vi "BluePlot Main.vi"(10 "Init options":T6={"UI visible?"=FALSE, "Update rate (ms)"=250, "visible sidebar?"=FALSE, "time to plot (init)"=600.0, "time to plot (max)"=inf, "config file start path"=path ""} {"time to plot (init)" format="%<%H:%M:%S>t"}, 11 "BluePlotHandle":refnum<class "BluePlotHandle.lvclass">) -> ()   [LabVIEW 2021, in "BluePlot.lvlib"]
uses:
  BluePlot.lvlib
  TypeDefs/Plot top row.ctl
  Classes/BluePlotHandle/BluePlotHandle.lvclass
  Classes/BluePlotHandle/SubVIs/Init Options.ctl
  TypeDefs/plot load data V2.ctl
  TypeDefs/plot properties V2.ctl
  TypeDefs/plot attributes V2.ctl
  TypeDefs/Plot scale axis properties.ctl
  TypeDefs/Plot general properties.ctl
  TypeDefs/plot event struc data.ctl
  TypeDefs/Plot active mode.ctl
  TypeDefs/Plot UI references.ctl
  TypeDefs/plot while loop data.ctl
  Classes/BluePlotHandle/BluePlotHandle.lvclass/BluePlotHandle.ctl
  SubVIs/autocomplete string/autocomplete key focus states.ctl
  TypeDefs/load config mode.ctl
  <vilib>/Utility/miscctls.llb/LVPointTypeDef.ctl
  TypeDefs/plot handle queue data.ctl
  TypeDefs/Plot QSM action.ctl
  <vilib>/Futures/Futures/Promise/Promise.lvclass
  TypeDefs/Save 1PLOT config.ctl
  <userlib>/Blue Origin/BlueSerialization/BlueSerializer/BlueSerializer.lvclass
  <userlib>/Blue Origin/BlueJSONTextSerializer/Classes/BlueJSONTextSerializer/BlueJSONTextSerializer.lvclass
  C:/Program Files/National Instruments/LabVIEW 2021/user.lib/Blue Origin/BlueSerialization/BlueSerializer/BlueSerializer.lvclass
panel:
  in  "Save 1PLOT (spoof)":bool
  in  "Load 1PLOT (spoof)":bool
  in  "Open Settings (spoof)":bool
  in  "clear plot config":bool
  in  "Load Plot config":T1={"plots"=[], "X-axis"={"Name Label.Text"="", "Style"=0, "Tick Colors:Minor Tick Color"=0, "Tick Colors:Tick Color"=0, "Marker Colors:Text Color"=0, "Grid Colors:Major Color"=0, "Grid Colors:Minor Color"=0, "Mapping Mode"=0, "Flipped"=FALSE, "Name Label.Visible"=FALSE, "Name Label.Text Colors:Text Color"=0, "Scale Fit"=0, "Editable"=FALSE, "Range:Maximum"=0.0, "Range:Minimum"=0.0, "Offset and Multiplier:Multiplier"=0.0, "Offset and Multiplier:Offset"=0.0, "Name Label.Font:Size"=0, "Marker.Font:Size"=0, "Uniform Marker Spacing?"=TRUE, "Format String"=""}, "Y-axes"=[], "General"={"Title"="", "Time to Plot"=1800.0, "Title.Visible"=FALSE, "Sidebar.Visible"=FALSE, "Plot Area:Colors:BG Color"=0}} {"General"."Time to Plot" format="%<%M:%S>t"}
  in  "Tab":enum32{"Page 1"}(tab)
  in  "Add row":bool
  in  "Time to Plot":dbl=1800.0 format="%<%H:%M:%S>t"
  in  "Title Visible?":bool
  in  "Splitter locked?":bool
  in  "Erase Plot":bool
  in  "Open Settings":bool
  in  "Save 1PLOT":bool
  in  "Load 1PLOT":bool
  out "Numerics":dbl[](array[numeric])
  in  "Scrollbar":i32(c297)
  in  "spoof1":T7(graph)
  out "dummy":bool
  in  "visible?":bool
  in  "top array":T8[](array[typedef])
  in  "Shutdown":bool
  in  "Title":string="Title"
  in  "visible sidebar?":bool
  out "Plot":cluster{"Timestamps":dbl[], "Data":dbl[]}[](graph)
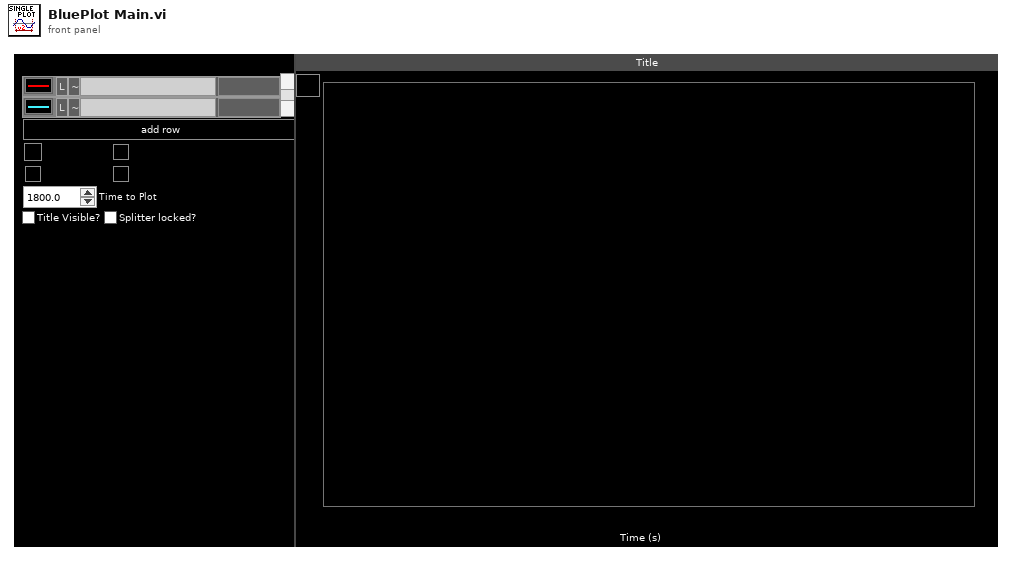
[diagram p1: front panel]
types:
  T1 = typedef "BluePlot.lvlib/plot load data V2.ctl" = cluster{"plots":T2[], "X-axis":T4, "Y-axes":T4[], "General":T5}
  T2 = typedef "BluePlot.lvlib/plot properties V2.ctl" = cluster{"attributes":T3, "Numeric":dbl, "Flatline?":bool}
  T3 = typedef "BluePlot.lvlib/plot attributes V2.ctl" = cluster{"Plot Color":u32, "Point Style":u8, "Line Style":u8, "Plot Interpolation":u8, "Line Width":u8, "Bar Plot Style":u8, "Fill To":i16, "X Scale Index":u32, "Y Scale Index":u32, "Anti-aliased":bool, "Label Format":u8, "Digital Transition Type":u8, "Digital Transition Location":u8, "Digital Line Style":u8, "Fill/Point Color":u32, "Plot Name":string, "Visible":bool}
  T4 = typedef "BluePlot.lvlib/Plot scale axis properties.ctl" = cluster{"Name Label.Text":string, "Style":u8, "Tick Colors:Minor Tick Color":u32, "Tick Colors:Tick Color":u32, "Marker Colors:Text Color":u32, "Grid Colors:Major Color":u32, "Grid Colors:Minor Color":u32, "Mapping Mode":u8, "Flipped":bool, "Name Label.Visible":bool, "Name Label.Text Colors:Text Color":u32, "Scale Fit":u8, "Editable":bool, "Range:Maximum":dbl, "Range:Minimum":dbl, "Offset and Multiplier:Multiplier":dbl, "Offset and Multiplier:Offset":dbl, "Name Label.Font:Size":u32, "Marker.Font:Size":u32, "Uniform Marker Spacing?":bool, "Format String":string}
  T5 = typedef "BluePlot.lvlib/Plot general properties.ctl" = cluster{"Title":string, "Time to Plot":dbl, "Title.Visible":bool, "Sidebar.Visible":bool, "Plot Area:Colors:BG Color":u32}
  T6 = typedef "BluePlot.lvlib/BluePlotHandle.lvclass/Init Options.ctl" = cluster{"UI visible?":bool, "Update rate (ms)":u32, "visible sidebar?":bool, "time to plot (init)":dbl, "time to plot (max)":dbl, "config file start path":path}
  T7 = cluster{cluster{"Time Stamp":dbl, "Data Value":dbl}[]}[]
  T8 = typedef "BluePlot.lvlib/Plot top row.ctl" = cluster{"PID":string, "index":i32, "PID color":u32, "right axis?":bool, "Flatline?":bool, "Numeric color":u32, "Data":string, "Flat":string}
  T9 = typedef "BluePlot.lvlib/plot while loop data.ctl" = cluster{"updating?":bool}
  T10 = typedef "BluePlot.lvlib/Plot UI references.ctl" = cluster{"Title":refnum<vi>, "Title?":refnum<vi>, "Visible sidebar?":refnum<vi>, "Time to Plot":refnum<vi>, "top array":refnum<vi>, "Scrollbar":refnum<vi>, "tab ref":refnum<vi>, "Add row":refnum<vi>, "TopArray":cluster{"PID":refnum<vi>, "Numeric color":refnum<vi>, "Flat":refnum<vi>, "PID color":refnum<vi>, "Data":refnum<vi>}, "Splitter":refnum<vi>, "splitter locked?":refnum<vi>, "Front Panel":refnum<vi>, "VI":refnum<vi>, "Meta LUT":refnum<data-value>, "Plot":refnum<vi>, "spoof":refnum<vi>, "BluePlotHandle":refnum<class "BluePlotHandle.lvclass">}
  T11 = typedef "BluePlot.lvlib/Plot active mode.ctl" = enum16{"inactive", "active PID", "active flatline"}
  T12 = typedef "BluePlot.lvlib/plot event struc data.ctl" = cluster{"Index":i32, "visible?":bool, "status":T11, "Event Reg":refnum<event-registration>, "All Names":string[]}
  T13 = typedef "BluePlot.lvlib/Plots listbox popout refs.ctl" = cluster{"VI":refnum<vi>, "Listbox":refnum<vi>, "font":cluster{"Font Name:":string, "Size":i16, "Strikeout?":bool, "Italic?":bool, "Underline?":bool, "Outline?":bool, "Shadow?":bool, "Bold?":bool}}
  T14 = typedef "BluePlot.lvlib/Save 1PLOT config.ctl" = cluster{"BlueSerializer":refnum<class "BlueSerializer.lvclass">, "file extension":string, "start path":path}
  T15 = enum16{"No Scaling", "Scale All Objects", "Scale Single Object"}
  T16 = cluster{"Color":u32, "PointStyle":u8, "LineStyle":u8, "Interp":u8, "LineWidth":u8, "BarPlotStyle":u8, "FillTo":i16, "XScaleIdx":u32, "YScaleIdx":u32, "Anti-Aliased":bool, "LabelFormat":u8, "TransitionType":u8, "TransitionLocation":u8, "DigitalLineStyle":u8}
  T17 = typedef "Plot top row.ctl" = cluster{"PID":string, "index":i32, "PID color":u32, "right axis?":bool, "Flatline?":bool, "Numeric color":u32, "Data":string, "Flat":string}
  T18 = typedef "BluePlot.lvlib/autocomplete key focus states.ctl" = enum16{"idle", "stop check", "start check"}
  T19 = typedef "BluePlot.lvlib/load config mode.ctl" = enum16{"Default (All)", "Init"}
  T20 = typedef "LVPositionTypeDef.ctl" = cluster{"Left":i32, "Top":i32}
  T21 = typedef "eventvkey.ctl" = enum16{"ASCII", "Enter", "Return", "Shift", "Ctrl", "Alt", "Cmd", "Opt", "Caps", "NumLock", "Clear", "Break", "Up", "Down", "Left", "Right", "Insert", "Delete", "Home", "End", "PageUp", "PageDown", "Escape", "Help", "Pause", "ScrollLock", "F1", "F2", "F3", "F4", "F5", "F6", "F7", "F8", "F9", "F10", "F11", "F12", "F13", "F14", "F15", "F16", "F17", "F18", "F19", "F20", "F21", "F22", "F23", "F24", "Play", "VolumeUp", "VolumeDown", "Mute", "Two Byte Char"}
  T22 = typedef "LVPoint32TypeDef.ctl" = cluster{"Horizontal":i32, "Vertical":i32}
  T23 = typedef "BluePlot.lvlib/Plot QSM action.ctl" = enum16{"start updating", "stop updating", "Shutdown", "Update", "Init", "Get Config", "Load Config"}
  T24 = typedef "BluePlot.lvlib/plot handle queue data.ctl" = cluster{"action":T23, "data":variant}
  T25 = typedef "LVPointTypeDef.ctl" = cluster{"Horizontal":i16, "Vertical":i16}
  T26 = typedef "BluePlot.lvlib/plot datapoint.ctl" = cluster{"Timestamps":dbl[], "Data":dbl[]}
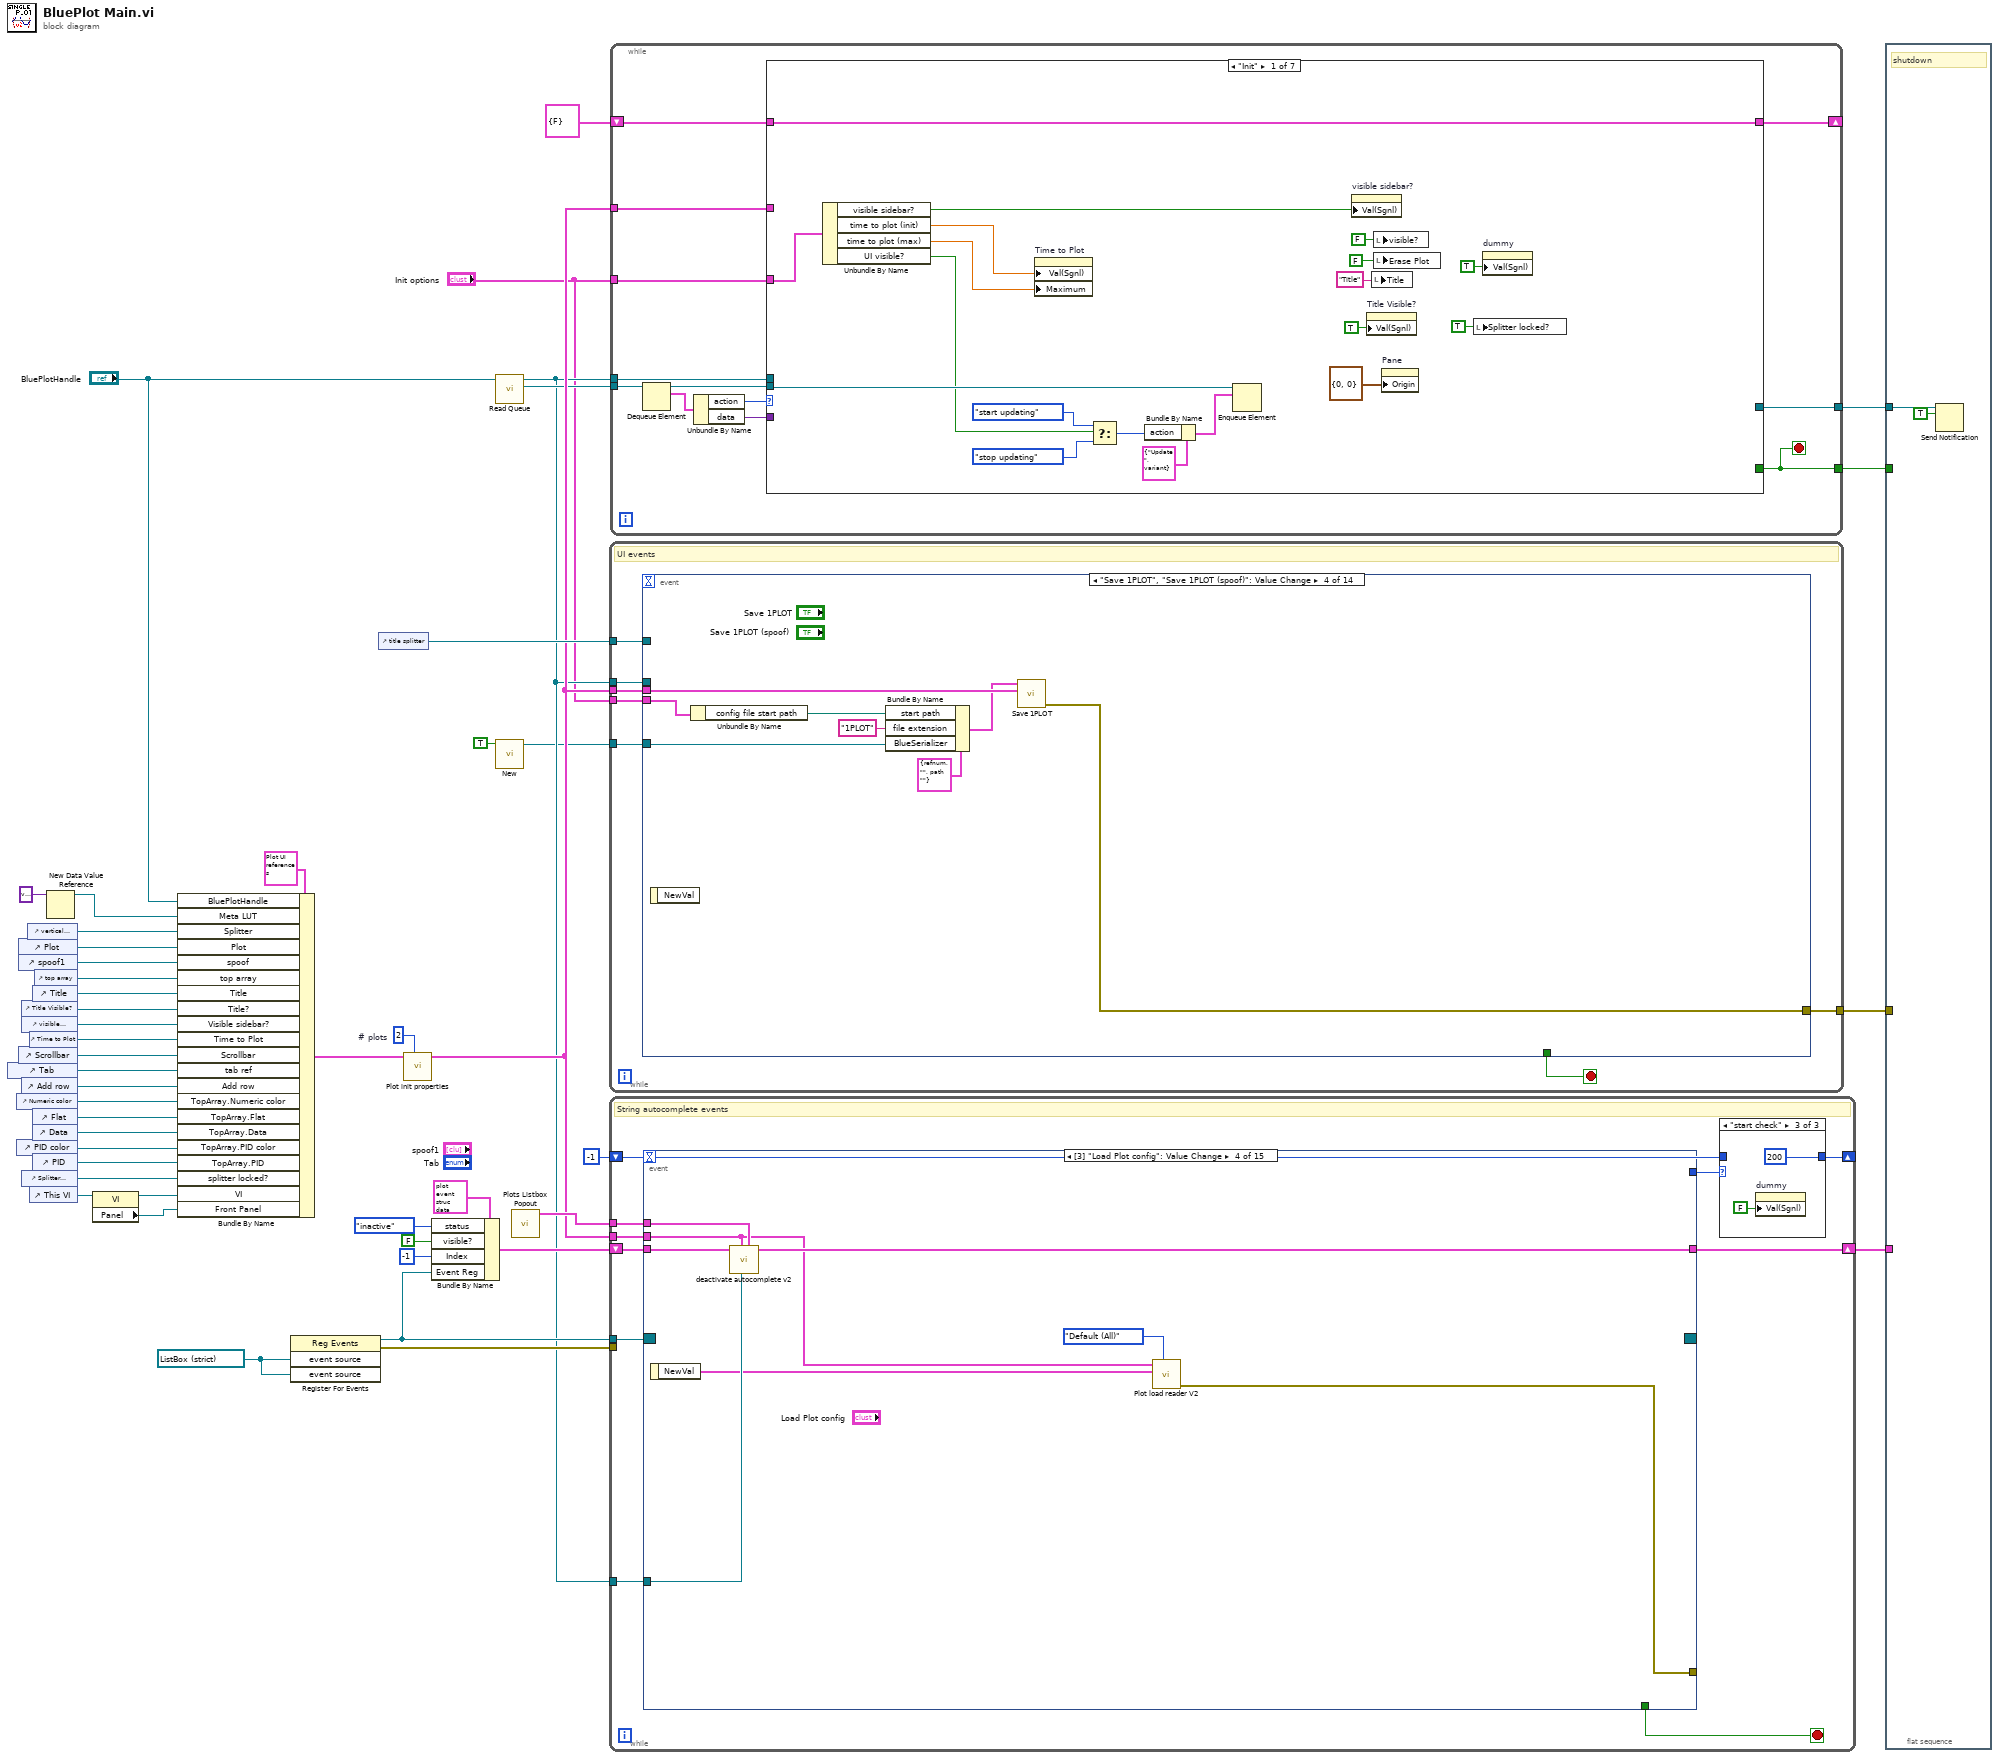
[diagram p0: block diagram]
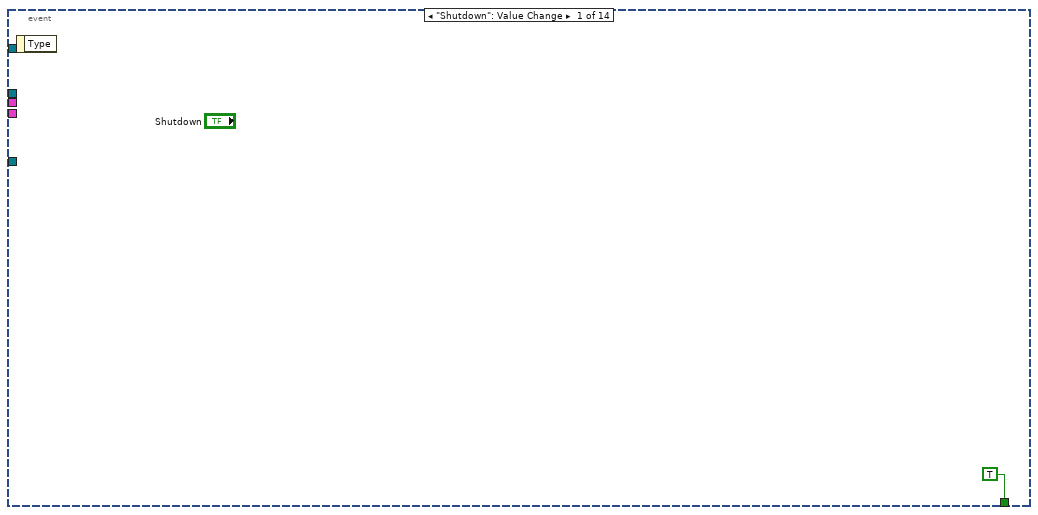
[diagram p2: hidden frame]
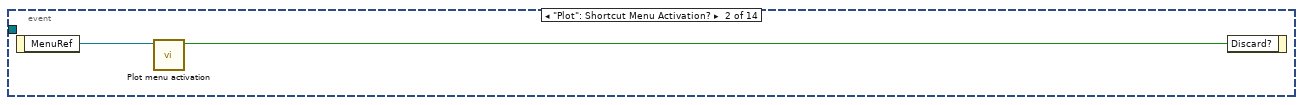
[diagram p3: hidden frame]
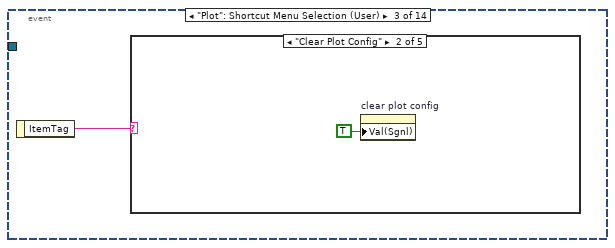
[diagram p4: hidden frame]
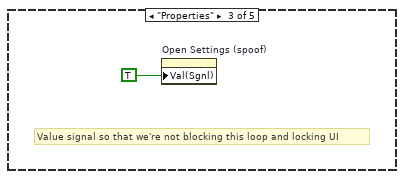
[diagram p6: hidden frame]
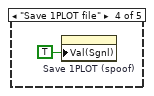
[diagram p7: hidden frame]
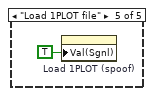
[diagram p8: hidden frame]
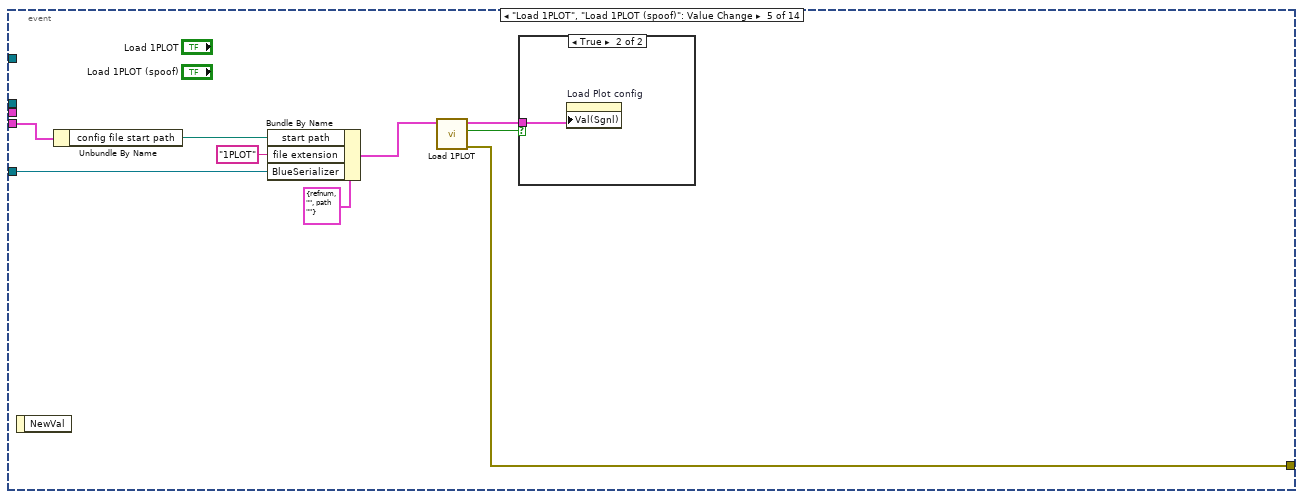
[diagram p9: hidden frame]
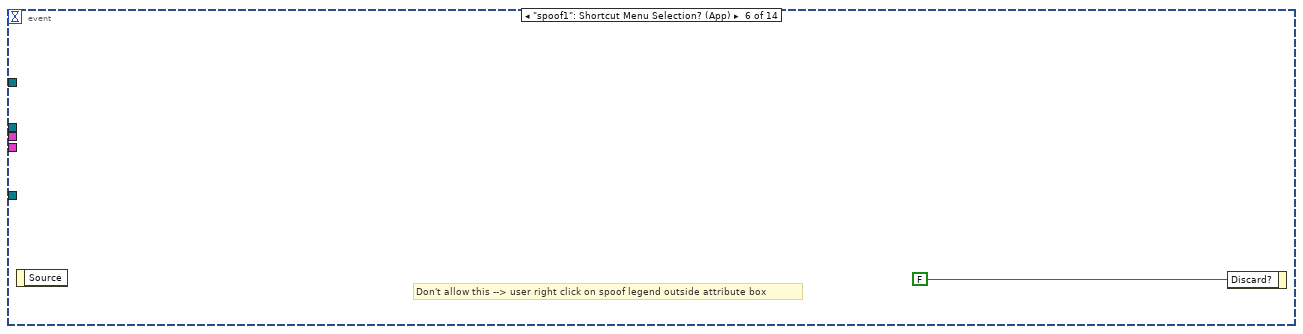
[diagram p11: hidden frame]
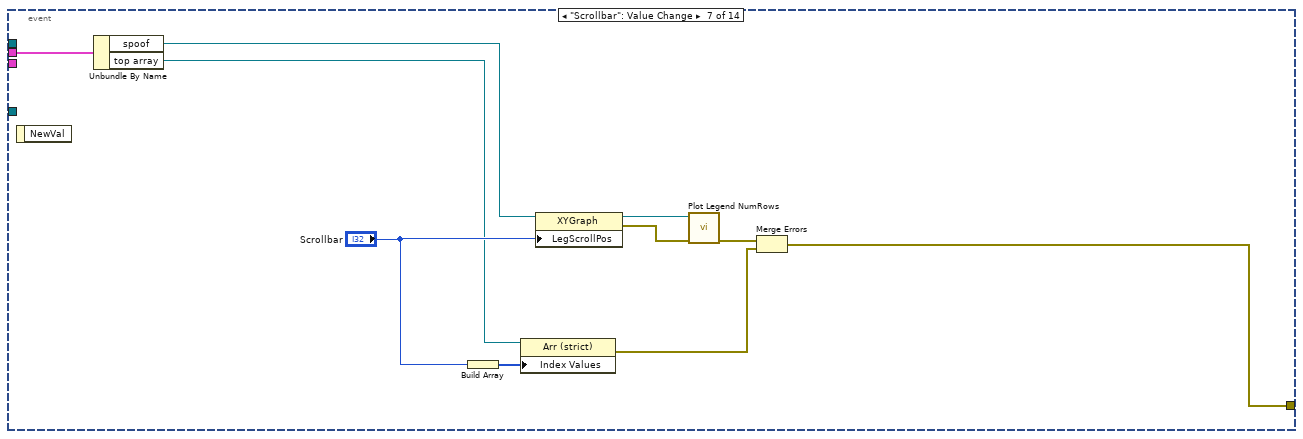
[diagram p12: hidden frame]
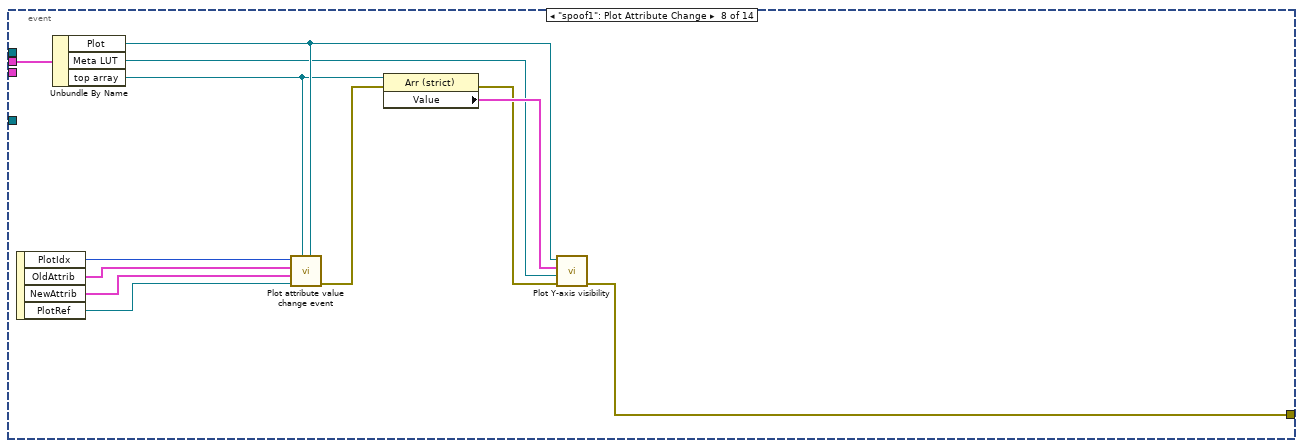
[diagram p13: hidden frame]
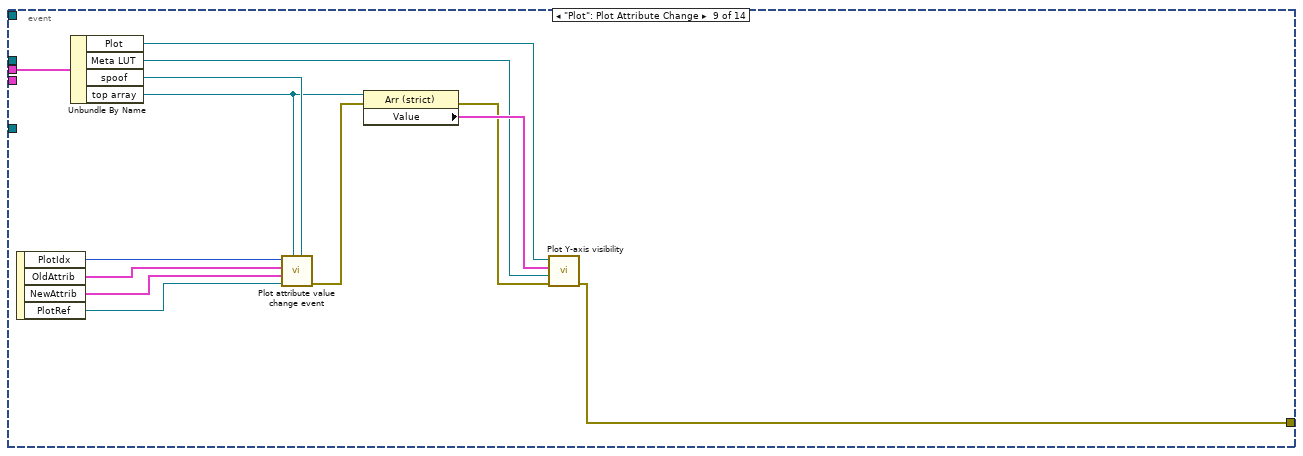
[diagram p14: hidden frame]
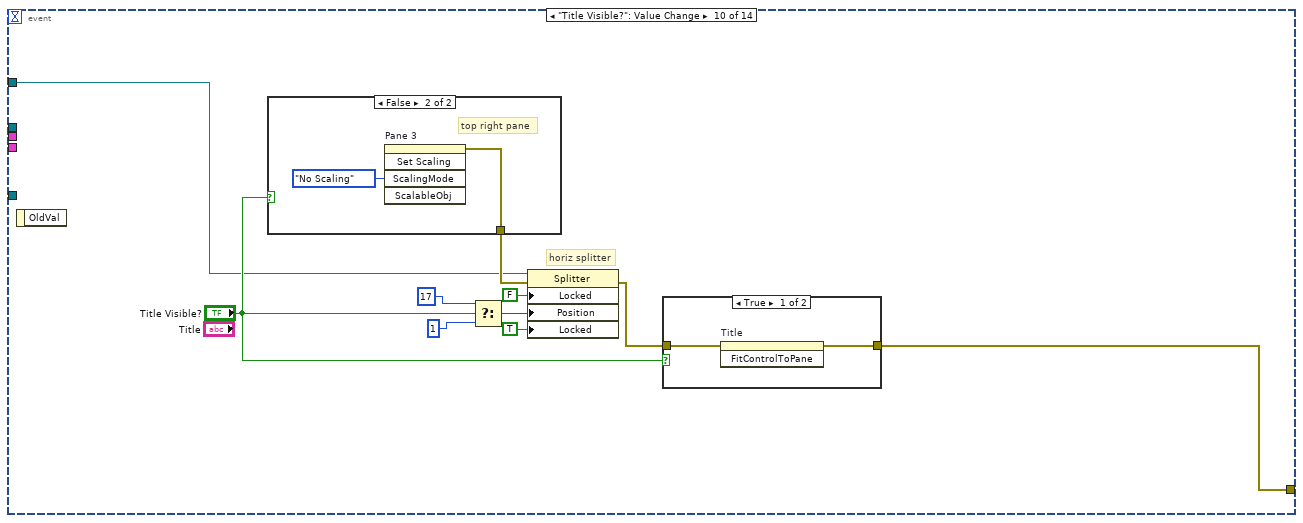
[diagram p15: hidden frame]
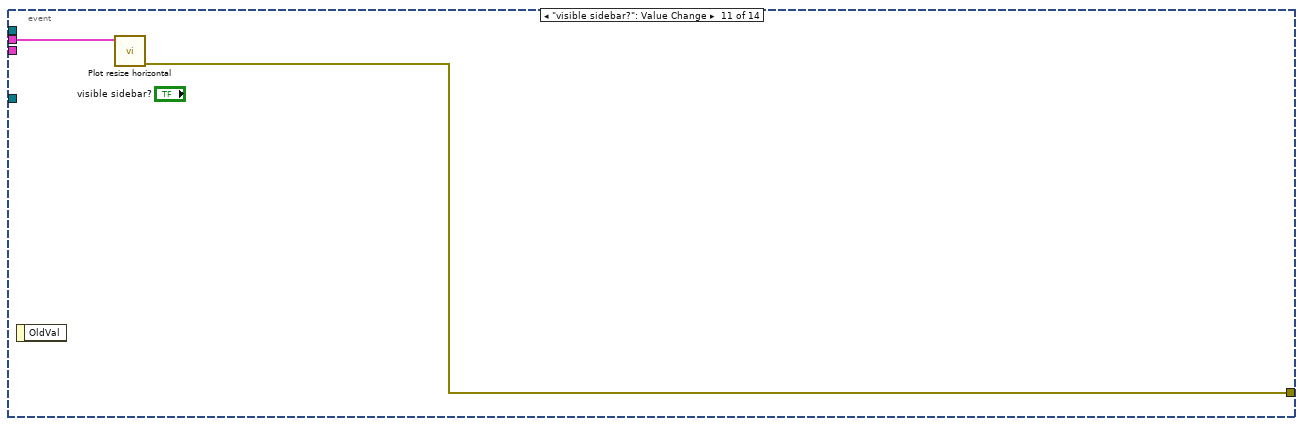
[diagram p18: hidden frame]
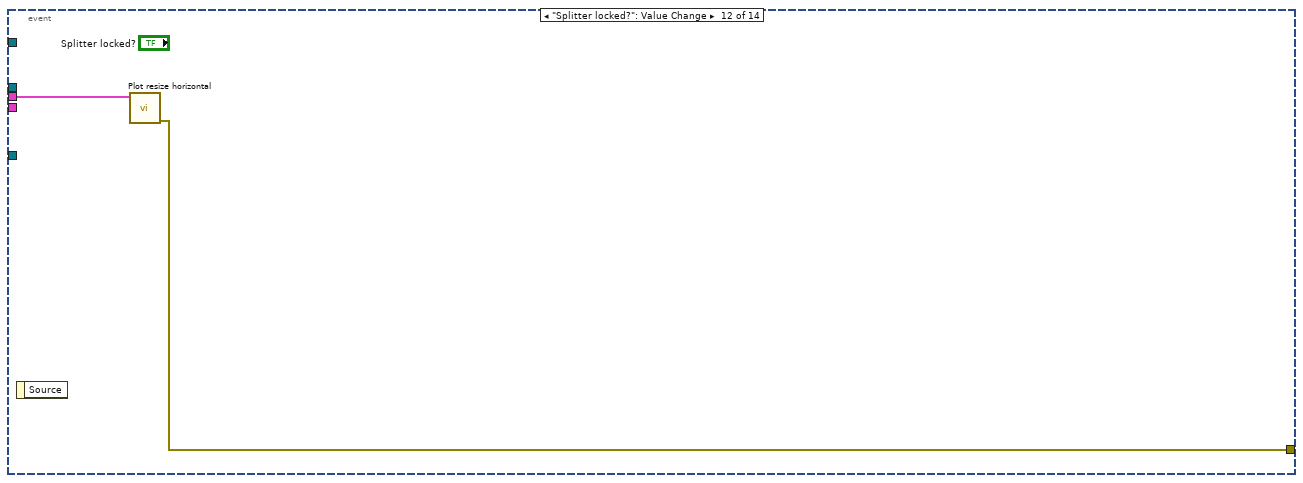
[diagram p19: hidden frame]
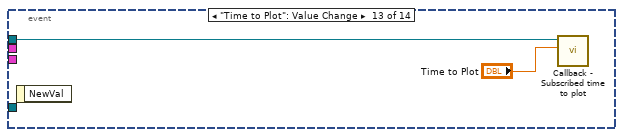
[diagram p20: hidden frame]
diagram:
  w20 = refnum<vi> refnum ("event source")
  w33 = 2  # # plots
  n1 = control-ref of="Tab"() -> (w34:refnum<vi>)
  n2 = control-ref of="Numeric color"() -> (w17:refnum<vi>)
  n3 = control-ref of="PID color"() -> (w14:refnum<vi>)
  n4 = control-ref of="Plot"() -> (w8:refnum<vi>)
  n5 = control-ref of="spoof1"() -> (w32:refnum<vi>)
  n6 = control-ref of="Scrollbar"() -> (w35:refnum<vi>)
  n7 = control-ref of="Title Visible?"() -> (w37:refnum<vi>)
  n8 = control-ref of="visible sidebar?"() -> (w4:refnum<vi>)
  n9 = control-ref of="Add row"() -> (w29:refnum<vi>)
  n10 = control-ref of="Splitter locked?"() -> (w26:refnum<vi>)
  n11 = control-ref of="vertical splitter"() -> (w27:refnum<vi>)
  n12 = control-ref of="Time to Plot"() -> (w38:refnum<vi>)
  n13 = control-ref of="This VI"() -> (w28:refnum<vi>)
  n14 = control-ref of="Title"() -> (w36:refnum<vi>)
  n15 = control-ref of="Flat"() -> (w16:refnum<vi>)
  n16 = control-ref of="Data"() -> (w15:refnum<vi>)
  n17 = control-ref of="PID"() -> (w21:refnum<vi>)
  n18 = control-ref of="top array"() -> (w31:refnum<vi>)
  n19 = New Data Value Reference(data value=variant) -> (data value reference=w12:refnum<data-value>)  [unwired: 1 in, 1 out]
  n20 = property class="VI"(reference=w28) -> (reference out=w22:refnum<vi>, "Panel"=w23:refnum<vi>)  [unwired: 1 in, 1 out]
  n21 = Bundle By Name(cluster=T10 {"Title"=refnum, "Title?"=refnum, "Visible sidebar?"=refnum, "Time to Plot"=refnum, "top array"=refnum, "Scrollbar"=refnum, "tab ref"=refnum, "Add row"=refnum, "TopArray"={"PID"=refnum, "Numeric color"=refnum, "Flat"=refnum, "PID color"=refnum, "Data"=refnum}, "Splitter"=refnum, "splitter locked?"=refnum, "Front Panel"=refnum, "VI"=refnum, "Meta LUT"=refnum, "Plot"=refnum, "spoof"=refnum, "BluePlotHandle"=refnum} ("Cluster"), "BluePlotHandle"="BluePlotHandle", "Meta LUT"=w12, "Splitter"=w27, "Plot"=w8, "spoof"=w32, "top array"=w31, "Title"=w36, "Title?"=w37, "Visible sidebar?"=w4, "Time to Plot"=w38, "Scrollbar"=w35, "tab ref"=w34, "Add row"=w29, "TopArray.Numeric color"=w17, "TopArray.Flat"=w16, "TopArray.Data"=w15, "TopArray.PID color"=w14, "TopArray.PID"=w21, "splitter locked?"=w26, "VI"=w22, "Front Panel"=w23) -> (w30:T10)
  n22 = register-events(w20, w20) -> (reference out=w19:refnum<event-registration>, error out=w18:errorcluster)  [unwired: 2 in]
  n23 = control-ref of="title splitter"() -> (w25:refnum<vi>)
  n24 = call "Plot init properties.vi"("# plots"=w33, "Refs"=w30) -> ("Refs (dup)"=w11:T10)  [unwired: 8 in, 1 out]
  n25 = Bundle By Name(cluster=T12 {"Index"=0, "visible?"=FALSE, "status"=enum."inactive", "Event Reg"=refnum, "All Names"=[]}, "status"=Plot_active_mode."inactive", "visible?"=FALSE ("active?"), "Index"=-1, "Event Reg"=w19) -> (w46:T12)
  n26 = call "Read Queue.vi"("BluePlotHandle in"="BluePlotHandle") -> ("Queue"=w10:refnum<queue>, "BluePlotHandle out"=w7:refnum<class "BluePlotHandle.lvclass">)  [unwired: 8 in, 1 out]
  n27 = call <userlib>:"New.vi"("PrettyPrint?"=TRUE) -> ("BlueJSONTextSerializer out"=w1:refnum<class "BlueJSONTextSerializer.lvclass">)  [unwired: 9 in, 1 out]
  n28 = call "Plots Listbox Popout.vi"() -> ("Refs"=w24:T13)  [unwired: 11 in]
  n29 = while {
    tunnel: [w52] -> w43
    tunnel: w11 -> [w54]
    tunnel: w25 -> [w53]
    tunnel: w7 -> [w51]
    tunnel: "Init options" -> [w50]
    tunnel: w1 -> [w49]
    stop <- w55 stop-if-true
    # "UI events"
    n30 = event shown="[3] \"Save 1PLOT\", \"Save 1PLOT (spoof)\": Value Change" {
      selector: _ -> [_ _ _ _ _ _ _ _ _ _ _ _ _ _]
      dyn-events: _ -> [_ _ _ _ _ _ _ _ _ _ _ _ _ _]
      timeout: _ -> [_ _ _ _ _ _ _ _ _ _ _ _ _ _]
      tunnel: [TRUE _ _ _ _ _ _ _ _ _ _ _ _ _] -> w55
      tunnel: [_ _ _ w70 w78 _ w86 w99 w112 w119 w133 w135 _ w139] -> w52
      tunnel: w54 -> [_ _ _ w71 _ _ w85 w98 w111 _ w134 w136 _ w140]
      tunnel: w53 -> [_ _ _ _ _ _ _ _ _ w118 _ _ _ _]
      tunnel: w51 -> [_ _ _ _ _ _ _ _ _ _ _ _ w138 _]
      tunnel: w50 -> [_ _ _ w67 w73 _ _ _ _ _ _ _ _ _]
      tunnel: w49 -> [_ _ _ w65 w74 _ _ _ _ _ _ _ _ _]
      event "Shutdown": Value Change {
        n31 = event-data() -> ()  [unwired: 1 in, 1 out]
      }
      event "Plot": Shortcut Menu Activation? {
        n32 = event-data() -> ("MenuRef"=w58:refnum<k9>)  [unwired: 1 in]
        n33 = call "Plot menu activation.vi"("MenuRef"=w58) -> ("Discard?"=w57:bool)  [unwired: 9 in, 1 out]
        n34 = event-data("Discard?"=w57) -> ()  [unwired: 1 in, 1 out]
      }
      event "Plot": Shortcut Menu Selection (User) {
        n35 = event-data() -> ("ItemTag"=w59:string)  [unwired: 1 in]
        n36 = case shown="\"Clear Plot Config\"" w59 {
          frame Default {
          }
          frame "Clear Plot Config" {
            n37 = property on="clear plot config" class="Bool (strict)"("Val(Sgnl)"=TRUE ("Value (Signaling)")) -> ()  [unwired: 2 in, 2 out]
          }
          frame "Properties" {
            # "Value signal so that we're not blocking this loop and locking UI"
            n38 = property on="Open Settings (spoof)" class="Bool (strict)"("Val(Sgnl)"=TRUE ("Value (Signaling)")) -> ()  [unwired: 2 in, 2 out]
          }
          frame "Save 1PLOT file" {
            n39 = property on="Save 1PLOT (spoof)" class="Bool (strict)"("Val(Sgnl)"=TRUE ("Value (Signaling)")) -> ()  [unwired: 2 in, 2 out]
          }
          frame "Load 1PLOT file" {
            n40 = property on="Load 1PLOT (spoof)" class="Bool (strict)"("Val(Sgnl)"=TRUE ("Value (Signaling)")) -> ()  [unwired: 2 in, 2 out]
          }
        }
      }
      event "Save 1PLOT", "Save 1PLOT (spoof)": Value Change {
        n41 = event-data() -> ()  [unwired: 1 in, 1 out]
        n42 = Unbundle By Name(w67) -> ("config file start path"=w66:path)
        n43 = Bundle By Name(cluster=T14 {"BlueSerializer"=refnum, "file extension"="", "start path"=path ""} ("Config Ops"), "start path"=w66, "file extension"="1PLOT", "BlueSerializer"=w65) -> (w64:T14)
        n44 = call "Save 1PLOT.vi"("Refs"=w71, "Config Ops"=w64) -> ("error out"=w70:errorcluster)  [unwired: 9 in]
      }
      event "Load 1PLOT", "Load 1PLOT (spoof)": Value Change {
        n45 = event-data() -> ()  [unwired: 1 in, 1 out]
        n46 = Unbundle By Name(w73) -> ("config file start path"=w77:path)
        n47 = Bundle By Name(cluster=T14 {"BlueSerializer"=refnum, "file extension"="", "start path"=path ""} ("Config Ops"), "start path"=w77, "file extension"="1PLOT", "BlueSerializer"=w74) -> (w72:T14)
        n48 = call "Load 1PLOT.vi"("Config Ops"=w72) -> ("error out"=w78:errorcluster, "Valid load?"=w79:bool, "Plot Config"=w80:T1)  [unwired: 8 in]
        n49 = case shown="True" w79 {
          tunnel: w80 -> [_ w81]
          frame False {
          }
          frame True {
            n50 = property on="Load Plot config" class="Clust (strict)"("Val(Sgnl)"=w81) -> ()  [unwired: 2 in, 2 out]
          }
        }
      }
      event "spoof1": Shortcut Menu Selection? (App) {
        # "Don't allow this --> user right click on spoof legend outside attribute box"
        n51 = event-data() -> ()  [unwired: 1 in, 1 out]
        n52 = event-data("Discard?"=FALSE) -> ()  [unwired: 1 in, 1 out]
      }
      event "Scrollbar": Value Change {
        n53 = event-data() -> ()  [unwired: 1 in, 1 out]
        n54 = Unbundle By Name(w85) -> ("spoof"=w83:refnum<vi>, "top array"=w84:refnum<vi>)
        n55 = Build Array("Scrollbar") -> (w92:i32[])
        n56 = property class="Arr (strict)"(reference=w84, "Index Values"=w92) -> (error out=w87:errorcluster)  [unwired: 1 in, 1 out]
        n57 = property class="XYGraph"(reference=w83, "LegScrollPos"="Scrollbar") -> (reference out=w91:refnum<vi>, error out=w90:errorcluster)  [unwired: 1 in]
        n58 = call "Plot Legend NumRows.vi"("error in (no error)"=w90, "XY graph ref"=w91) -> ("error out"=w88:errorcluster)  [unwired: 8 in, 1 out]
        n59 = Merge Errors(w88, w87) -> (w86:errorcluster)
      }
      event "spoof1": Plot Attribute Change {
        n60 = event-data() -> ("PlotIdx"=w104:i32, "OldAttrib"=w103:T16, "NewAttrib"=w102:T16, "PlotRef"=w101:refnum<vi>)  [unwired: 1 in]
        n61 = Unbundle By Name(w98) -> ("Plot"=w97:refnum<vi>, "Meta LUT"=w96:refnum<data-value>, "top array"=w95:refnum<vi>)
        n62 = call "Plot attribute value change event.vi"("Plot ref (target)"=w97, "top array"=w95, "PlotRef (event source)"=w101, "NewAttrib"=w102, "OldAttrib"=w103, "PlotIdx (target)"=w104) -> ("error out"=w94:errorcluster)  [unwired: 5 in]
        n63 = property class="Arr (strict)"(reference=w95, error in=w94) -> (error out=w93:errorcluster, "Value"=w100:T17[])  [unwired: 1 out]
        n64 = call "Plot Y-axis visibility.vi"("error in (no error)"=w93, "Meta LUT"=w96, "top array"=w100, "Plot"=w97) -> ("error out"=w99:errorcluster)  [unwired: 7 in]
      }
      event "Plot": Plot Attribute Change {
        n65 = event-data() -> ("PlotIdx"=w116:i32, "OldAttrib"=w114:T16, "NewAttrib"=w115:T16, "PlotRef"=w117:refnum<vi>)  [unwired: 1 in]
        n66 = Unbundle By Name(w111) -> ("Plot"=w110:refnum<vi>, "Meta LUT"=w108:refnum<data-value>, "spoof"=w109:refnum<vi>, "top array"=w107:refnum<vi>)
        n67 = call "Plot attribute value change event.vi"("Plot ref (target)"=w109, "top array"=w107, "PlotRef (event source)"=w117, "NewAttrib"=w115, "OldAttrib"=w114, "PlotIdx (target)"=w116) -> ("error out"=w106:errorcluster)  [unwired: 5 in]
        n68 = property class="Arr (strict)"(reference=w107, error in=w106) -> (error out=w105:errorcluster, "Value"=w113:T17[])  [unwired: 1 out]
        n69 = call "Plot Y-axis visibility.vi"("error in (no error)"=w105, "Meta LUT"=w108, "top array"=w113, "Plot"=w110) -> ("error out"=w112:errorcluster)  [unwired: 7 in]
      }
      event "Title Visible?": Value Change {
        # "horiz splitter"
        n70 = event-data() -> ()  [unwired: 1 in, 1 out]
        n71 = case shown="False" "Title Visible?" {
          tunnel: [_ w131] -> w122
          frame True {
          }
          frame False {
            # "top right pane"
            n72 = invoke on="Pane 3" class="Pane" method="Set Scaling"("ScalingMode"=T15."No Scaling" ("Scaling Mode")) -> (error out=w131:errorcluster)  [unwired: 4 in, 4 out]
          }
        }
        n73 = Select(t=17 ("Splitter Position"), s="Title Visible?", f=1 ("Splitter Position")) -> (s? t:f=w124:i32)
        n74 = property on="Property Node" class="Splitter"(reference=w118, error in=w122, "Locked"=FALSE ("Splitter Position Locked"), "Position"=w124, "Locked"=TRUE ("Splitter Position Locked")) -> (error out=w120:errorcluster)  [unwired: 1 out]
        n75 = case shown="True" "Title Visible?" {
          tunnel: w120 -> [w129 w130]
          tunnel: [w128 w130] -> w119
          frame True {
            n76 = invoke on="Title" class="Str" method="FitControlToPane"(error in=w129) -> (error out=w128:errorcluster)  [unwired: 2 in, 2 out]
          }
          frame False {
          }
        }
      }
      event "visible sidebar?": Value Change {
        n77 = event-data() -> ()  [unwired: 1 in, 1 out]
        n78 = call "Plot resize horizontal.vi"("Refs"=w134) -> ("error out"=w133:errorcluster)  [unwired: 10 in]
      }
      event "Splitter locked?": Value Change {
        n79 = event-data() -> ()  [unwired: 1 in, 1 out]
        n80 = call "Plot resize horizontal.vi"("Refs"=w136) -> ("error out"=w135:errorcluster)  [unwired: 10 in]
      }
      event "Time to Plot": Value Change {
        n81 = event-data() -> ()  [unwired: 1 in, 1 out]
        n82 = call-dynamic "Callback - Subscribed time to plot.vi"("time to plot (s)"="Time to Plot", "BluePlotHandle in"=w138) -> ()  [unwired: 8 in, 2 out]
      }
      event Pane Size {
        n83 = event-data() -> ()  [unwired: 1 in, 1 out]
        n84 = call "Plot resize vertical.vi"("Refs"=w140) -> ("error out"=w141:errorcluster)  [unwired: 8 in, 2 out]
        n85 = call "Plot resize horizontal.vi"("error in (no error)"=w141, "Refs"=w140) -> ("error out"=w139:errorcluster)  [unwired: 9 in]
      }
    }
  }
  n86 = while {
    tunnel: w24 -> [w150]
    shift-right: [w148] -> w42
    shift-left: w46 -> [w149]
    shift-right: [w147] -> _
    shift-left: -1 -> [w146]
    tunnel: w7 -> [w144]
    tunnel: w11 -> [w143]
    tunnel: w19 -> [w142]
    tunnel: w18 -> [_]
    stop <- w151 stop-if-true
    # "String autocomplete events"
    n87 = event shown="[3] \"Load Plot config\": Value Change" {
      selector: w142 -> [_ _ _ _ _ _ _ _ _ _ _ _ _ _ _]
      dyn-events: [w156 _ _ _ _ _ w233 _ _ _ w296 w305 _ w361 w373] -> _
      timeout: w146 -> [_ _ _ _ _ _ _ _ _ _ _ _ _ _ _]
      tunnel: [_ _ _ _ _ TRUE _ _ _ _ _ _ _ _ _] -> w151
      tunnel: w150 -> [w158 _ w190 w212 w219 w223 w230 _ w286 _ w298 w307 w331 w362 w375]
      tunnel: w149 -> [w161 w187 w198 w213 w220 w228 w243 w274 w291 w292 w304 w311 w333 w367 w380]
      tunnel: [w157 w187 w193 w210 w217 w226 w234 w273 w290 w292 w297 w306 w332 w360 w374] -> w148
      tunnel: [w163 _ w188 w208 w215 _ w231 _ w289 _ w302 w315 w329 w364 w377] -> _
      tunnel: [_ _ w195 _ _ _ _ _ _ _ _ _ _ _ _] -> w145
      tunnel: w144 -> [w160 _ w189 w211 w218 w224 w238 w272 _ _ w300 w310 _ w366 w379]
      tunnel: w143 -> [w159 _ w191 w209 w216 w227 w236 _ w288 _ w299 w309 _ w363 w376]
      event Timeout {
        n88 = event-data() -> ()  [unwired: 1 in, 1 out]
        n89 = Unbundle By Name(w161) -> ("status"=w162:T11)
        n90 = case shown="\"active PID\", \"active flatline\"" w162 {
          tunnel: [w166 w176] -> w163
          tunnel: w161 -> [w168 w175]
          tunnel: [w168 w174] -> w157
          tunnel: w160 -> [_ w173]
          tunnel: w159 -> [w165 w170]
          tunnel: w158 -> [_ w171]
          frame "inactive" {
            n91 = local read "Numerics"() -> (w167:dbl[])
            n92 = Unbundle By Name(w165) -> ("top array"=w164:refnum<vi>)
            n93 = call "Plot update numeric array.vi"("top array"=w164, "Numerics"=w167) -> ("error out"=w166:errorcluster)  [unwired: 9 in]
          }
          frame "active PID", "active flatline" {
            n94 = Unbundle By Name(w170) -> ("TopArray.PID"=w169:refnum<vi>)
            n95 = Unbundle By Name(w171) -> ("Listbox"=w172:refnum<vi>)
            n96 = property class="LstBox (strict)"(reference=w172) -> ("Key Focus"=w179:bool)  [unwired: 1 in, 2 out]
            n97 = property class="Str"(reference=w169) -> ("Key Focus"=w178:bool)  [unwired: 1 in, 2 out]
            n98 = Or(x=w179, y=w178) -> (x .or. y?=w177:bool)
            n99 = case shown="False" w177 {
              tunnel: [w183 _] -> w176
              tunnel: w175 -> [w185 w186]
              tunnel: [w184 w186] -> w174
              tunnel: w173 -> [w182 _]
              tunnel: w170 -> [w181 _]
              tunnel: w171 -> [w180 _]
              frame False {
                n100 = call "deactivate autocomplete v2.vi"("Listbox Refs"=w180, "BluePlotHandle"=w182, "Refs"=w181, "Loop data"=w185) -> ("error out"=w183:errorcluster, "Loop data"=w184:T12)  [unwired: 5 in, 1 out]
              }
              frame True {
              }
            }
          }
        }
        n101 = Unbundle By Name(w157) -> ("Event Reg"=w156:refnum<event-registration>)
      }
      event "dummy": Value Change {
        # "Fire this event to register timeout input"
        n102 = event-data() -> ()  [unwired: 1 in, 1 out]
      }
      event "visible?": Value Change {
        n103 = event-data() -> ()  [unwired: 1 in, 1 out]
        n104 = Bundle By Name(cluster=w198, "visible?"="visible?") -> (w194:T12)
        n105 = Select(t=autocomplete_key_focus_states."start check", s="visible?", f=autocomplete_key_focus_states."stop check") -> (s? t:f=w195:T18)
        n106 = case shown="False" "visible?" {
          tunnel: w194 -> [w204 w205]
          tunnel: [w203 w205] -> w193
          tunnel: w191 -> [w202 _]
          tunnel: w190 -> [w201 _]
          tunnel: w189 -> [w200 _]
          tunnel: [w199 _] -> w188
          frame False {
            n107 = call "deactivate autocomplete v2.vi"("Listbox Refs"=w201, "BluePlotHandle"=w200, "Refs"=w202, "Loop data"=w204) -> ("error out"=w199:errorcluster, "Loop data"=w203:T12)  [unwired: 5 in, 1 out]
          }
          frame True {
          }
        }
      }
      event Value Change {
        n108 = event-data() -> ("NewVal"=w207:T1)  [unwired: 1 in]
        n109 = call "deactivate autocomplete v2.vi"("Listbox Refs"=w212, "BluePlotHandle"=w211, "Refs"=w209, "Loop data"=w213) -> ("Loop data"=w210:T12)  [unwired: 5 in, 2 out]
        n110 = call "Plot load reader V2.vi"("Load Mode"=load_config_mode."Default (All)", "Plot config"=w207, "Refs"=w209) -> ("error out"=w208:errorcluster)  [unwired: 8 in]
      }
      event "clear plot config": Value Change {
        w214 = 2  # # plots
        n111 = event-data() -> ()  [unwired: 1 in, 1 out]
        n112 = call "deactivate autocomplete v2.vi"("Listbox Refs"=w219, "BluePlotHandle"=w218, "Refs"=w216, "Loop data"=w220) -> ("Loop data"=w217:T12)  [unwired: 5 in, 2 out]
        n113 = call "Plot init properties.vi"("# plots"=w214, "Refs"=w216) -> ("error out"=w215:errorcluster)  [unwired: 8 in, 1 out]
      }
      event "Shutdown": Value Change {
        n114 = event-data() -> ()  [unwired: 1 in, 1 out]
        n115 = call "deactivate autocomplete v2.vi"("Listbox Refs"=w223, "BluePlotHandle"=w224, "Refs"=w227, "Loop data"=w228) -> ("error out"=w225:errorcluster, "Loop data"=w226:T12)  [unwired: 5 in, 1 out]
        n116 = call <vilib>:"Clear Errors.vi"("error in (no error)"=w225) -> ()  [unwired: 5 in, 2 out]
        n117 = Unbundle By Name(w223) -> ("VI"=w222:refnum<vi>)
        n118 = invoke class="VI" method="FP.Close"(reference=w222) -> (error out=w221:errorcluster)  [unwired: 2 in, 2 out]
        n119 = call <vilib>:"Clear Errors.vi"("error in (no error)"=w221) -> ()  [unwired: 5 in, 2 out]
      }
      event "top array": Mouse Down {
        n120 = event-data() -> ()  [unwired: 1 in, 1 out]
        n121 = Unbundle By Name(w236) -> ("top array"=w235:refnum<vi>, "TopArray.PID"=w232:refnum<vi>)
        n122 = call "Array Point to RowCol V3.vi"("PID"=w232, "top array"=w235) -> ("error out"=w242:errorcluster, "Array Element.Position"=w240:T20, "Index"=w241:i32, "PID key focus?"=w239:bool, "Flatline?"=w237:bool)  [unwired: 5 in]
        n123 = case shown="True" w239 {
          tunnel: w243 -> [w245 w255]
          tunnel: w242 -> [w244 w257]
          tunnel: w230 -> [_ w256]
          tunnel: [w245 w252] -> w234
          tunnel: w240 -> [_ w250]
          tunnel: w241 -> [_ w251]
          tunnel: [w244 w249] -> w231
          tunnel: w238 -> [_ w248]
          tunnel: w237 -> [_ w247]
          tunnel: w236 -> [_ w246]
          frame False {
          }
          frame True {
            n124 = Unbundle By Name(w255) -> ("Index"=w254:i32)
            n125 = Equal?(x=w254, y=w251) -> (x = y?=w253:bool)
            n126 = case shown="False" w253 {
              tunnel: w257 -> [w269 w270]
              tunnel: w256 -> [w258 _]
              tunnel: w255 -> [w268 w271]
              tunnel: [w262 w271] -> w252
              tunnel: w251 -> [w261 _]
              tunnel: w250 -> [w260 _]
              tunnel: [w264 w270] -> w249
              tunnel: w248 -> [w267 _]
              tunnel: w247 -> [w259 _]
              tunnel: w246 -> [w263 _]
              frame False {
                n127 = call "deactivate autocomplete v2.vi"("Listbox Refs"=w258, "BluePlotHandle"=w267, "Refs"=w263, "error in (no error)"=w269, "Loop data"=w268) -> ("error out"=w265:errorcluster, "Loop data"=w266:T12)  [unwired: 4 in, 1 out]
                n128 = call "activate autocomplete v2.vi"("Listbox Refs"=w258, "Flatline?"=w259, "Refs"=w263, "error in (no error)"=w265, "Array Element.Position"=w260, "Index"=w261, "Loop data"=w266) -> ("error out"=w264:errorcluster, "Loop data"=w262:T12)  [unwired: 3 in]
              }
              frame True {
              }
            }
          }
        }
        n129 = Unbundle By Name(w234) -> ("Event Reg"=w233:refnum<event-registration>)
      }
      event "top array": Mouse Enter {
        n130 = event-data() -> ()  [unwired: 1 in, 1 out]
        n131 = in-place {
          in-place-border: w272 -> [w275]
          n132 = in-place-cluster #1(w274) -> ("status"=w279:T11, "All Names"=w276:string[])
          n133 = case shown="\"inactive\"" w279 {
            selector: w279 -> [w281 w284]
            tunnel: [w281 w284] -> w278
            tunnel: [w280 w283] -> w277
            tunnel: w276 -> [w280 _]
            tunnel: w275 -> [_ w282]
            frame "active PID", "active flatline" {
            }
            frame "inactive" {
              n134 = call-dynamic "Callback - Get Plottable Names.vi"("BluePlotHandle in"=w282) -> ("Plottable Names"=w283:string[])  [unwired: 8 in, 2 out]
            }
          }
          n135 = in-place-cluster #1("status"=w278, "All Names"=w277) -> (w273:T12)
        }
      }
      event "top array": Value Change {
        n136 = event-data() -> ("NewVal"=w285:T8[], "OldVal"=w287:T8[])  [unwired: 1 in]
        n137 = call "Plot TopArray ValueChange.vi"("Listbox Refs"=w286, "Refs"=w288, "OldVal"=w287, "NewVal"=w285, "Loop data"=w291) -> ("error out"=w289:errorcluster, "Loop data"=w290:T12)  [unwired: 5 in]
      }
      event "top array": Mouse Down? {
        n138 = event-data() -> ("Button"=w294:u16)  [unwired: 1 in]
        n139 = case shown="Default" w294 {
          tunnel: [_ TRUE] -> w293
          frame Default {
          }
          frame 2 {
            # "ignore right clicks"
          }
        }
        n140 = event-data("Discard?"=w293) -> ()  [unwired: 1 in, 1 out]
      }
      event Key Down? {
        n141 = event-data() -> ("VKey"=w303:T21)  [unwired: 1 in]
        n142 = call "Plot UpDown Vkey.vi"("BluePlotHandle"=w300, "Listbox Refs"=w298, "VKey"=w303, "Refs"=w299, "Loop data"=w304) -> ("error out"=w302:errorcluster, "Discard?"=w301:bool, "Loop data"=w297:T12)  [unwired: 4 in]
        n143 = Unbundle By Name(w297) -> ("Event Reg"=w296:refnum<event-registration>)
        n144 = event-data("Discard?"=w301) -> ()  [unwired: 1 in, 1 out]
      }
      event Mouse Down {
        n145 = event-data() -> ("Coords"=w316:T22)  [unwired: 1 in]
        n146 = Unbundle By Name(w307) -> ("Listbox"=w308:refnum<vi>)
        n147 = invoke class="LstBox (strict)" method="Point To Row"(reference=w308, "Point"=w316) -> (reference out=w313:refnum<vi>, error out=w312:errorcluster, "InBounds"=w314:bool)  [unwired: 5 in, 4 out]
        n148 = case shown="True" w314 {
          tunnel: w313 -> [w321 _]
          tunnel: w312 -> [w319 w326]
          tunnel: [w318 w325] -> w315
          tunnel: w311 -> [w317 w328]
          tunnel: [w317 w327] -> w306
          tunnel: w310 -> [_ w324]
          tunnel: w309 -> [_ w323]
          tunnel: w307 -> [_ w322]
          frame False {
            # "Don't lose focus young jedi"
            n149 = property class="LstBox (strict)"(reference=w321, error in=w319, "Key Focus"=TRUE) -> (error out=w318:errorcluster)  [unwired: 1 out]
          }
          frame True {
            n150 = call "deactivate autocomplete v2.vi"("Listbox Refs"=w322, "BluePlotHandle"=w324, "Refs"=w323, "error in (no error)"=w326, "Loop data"=w328) -> ("error out"=w325:errorcluster, "Loop data"=w327:T12)  [unwired: 4 in, 1 out]
          }
        }
        n151 = Unbundle By Name(w306) -> ("Event Reg"=w305:refnum<event-registration>)
      }
      event Mouse Move {
        n152 = event-data() -> ("Coords"=w330:T22)  [unwired: 1 in]
        n153 = in-place {
          in-place-border: w331 -> [w337]
          in-place-border: w330 -> [w335]
          in-place-border: [w334] -> w329
          n154 = in-place-cluster #2(w333) -> ("status"=w338:T11)
          n155 = case shown="\"active PID\"" w338 {
            selector: w338 -> [w339 w350]
            tunnel: w337 -> [_ w341]
            tunnel: [w339 w350] -> w336
            tunnel: w335 -> [_ w344]
            tunnel: [_ w342] -> w334
            frame "inactive", "active flatline" {
            }
            frame "active PID" {
              n156 = Unbundle By Name(w341) -> ("Listbox"=w340:refnum<vi>)
              n157 = invoke class="LstBox (strict)" method="Point To Row"(reference=w340, "Point"=w344) -> (reference out=w345:refnum<vi>, error out=w343:errorcluster, "Row"=w348:i32)  [unwired: 5 in, 4 out]
              n158 = feedback #3(-3 ("Row")) -> (w347:i32)
              n159 = feedback-in #3(w348) -> ()
              n160 = Not Equal?(x=w348, y=w347) -> (x != y?=w349:bool)
              n161 = case shown="True" w349 {
                tunnel: w345 -> [_ w355]
                tunnel: w348 -> [_ w354]
                tunnel: w343 -> [w351 w353]
                tunnel: [w351 w352] -> w342
                frame False {
                }
                frame True {
                  n162 = property class="LstBox (strict)"(reference=w355, error in=w353, "Active Row"=-2 ("Active Row:Active Row Number"), "CellBG"=u32 16448250, "Active Row"=w354, "CellBG"=u32 7465727) -> (error out=w352:errorcluster)  [unwired: 1 out]
                }
              }
            }
          }
          n163 = in-place-cluster #2("status"=w336) -> (w332:T12)
        }
      }
      event "Add row": Value Change {
        n164 = event-data() -> ()  [unwired: 1 in, 1 out]
        n165 = call "deactivate autocomplete v2.vi"("Listbox Refs"=w362, "BluePlotHandle"=w366, "Refs"=w363, "Loop data"=w367) -> ("error out"=w365:errorcluster, "Row added?"=w359:bool, "Loop data"=w360:T12)  [unwired: 5 in]
        n166 = case shown="False" w359 {
          tunnel: w365 -> [w371 w372]
          tunnel: [w369 w372] -> w364
          tunnel: w363 -> [w368 _]
          frame False {
            n167 = call "Plot add row.vi"("Refs"=w368, "error in (no error)"=w371) -> ("error out"=w370:errorcluster)  [unwired: 9 in]
            n168 = call "Plot resize vertical.vi"("error in (no error)"=w370, "Refs"=w368) -> ("error out"=w369:errorcluster)  [unwired: 7 in, 2 out]
          }
          frame True {
          }
        }
        n169 = Unbundle By Name(w360) -> ("Event Reg"=w361:refnum<event-registration>)
      }
      event "Open Settings (spoof)", "Open Settings": Value Change {
        n170 = event-data() -> ()  [unwired: 1 in, 6 out]
        n171 = call "deactivate autocomplete v2.vi"("Listbox Refs"=w375, "BluePlotHandle"=w379, "Refs"=w376, "Loop data"=w380) -> ("error out"=w378:errorcluster, "Loop data"=w374:T12)  [unwired: 5 in, 1 out]
        n172 = call "Plot Scales GUI V2.vi"("error in (no error)"=w378, "Refs"=w376) -> ("error out"=w377:errorcluster)  [unwired: 9 in]
        n173 = Unbundle By Name(w374) -> ("Event Reg"=w373:refnum<event-registration>)
      }
    }
    n174 = case shown="\"start check\"" w145 {
      tunnel: [w152 -1 200] -> w147
      tunnel: w146 -> [w152 _ _]
      frame "idle" {
      }
      frame "stop check" {
      }
      frame "start check" {
        n175 = property on="dummy" class="Bool (strict)"("Val(Sgnl)"=FALSE ("Value (Signaling)")) -> ()  [unwired: 2 in, 2 out]
      }
    }
  }
  n176 = while {
    tunnel: w10 -> [w392]
    tunnel: [w390] -> w44
    tunnel: w11 -> [w389]
    tunnel: "Init options" -> [w385]
    shift-right: [w382] -> _
    shift-left: T9 {"updating?"=FALSE} ("Cluster") -> [w384]
    tunnel: w7 -> [w383]
    tunnel: [w381] -> w5
    stop <- w390 stop-if-true
    n177 = Dequeue Element(queue=w392) -> (queue out=w391:refnum<queue>, element=w388:T24)  [unwired: 2 in, 2 out]
    n178 = Unbundle By Name(w388) -> ("action"=w387:T23, "data"=w386:variant)
    n179 = case shown="\"Init\"" w387 {
      tunnel: w391 -> [w409 w414 _ w427 _ _ w478]
      tunnel: [_ _ _ _ _ _ TRUE] -> w390
      tunnel: w389 -> [_ _ _ _ w454 _ w476]
      tunnel: w386 -> [_ _ _ _ w453 w467 w471]
      tunnel: w385 -> [w410 _ _ w429 _ _ _]
      tunnel: w384 -> [w408 w413 w424 w425 w450 w465 w474]
      tunnel: w383 -> [_ _ _ w426 _ _ _]
      tunnel: [w408 w412 w422 w425 w450 w465 w474] -> w382
      tunnel: [_ _ _ _ _ _ w469] -> w381
      frame "Init" {
        n180 = Unbundle By Name(w410) -> ("visible sidebar?"=w399:bool, "time to plot (init)"=w401:dbl, "time to plot (max)"=w400:dbl, "UI visible?"=w407:bool)
        n181 = property on="Time to Plot" class="DigNum (strict)"("Val(Sgnl)"=w401, "Maximum"=w400) -> ()  [unwired: 2 in, 2 out]
        n182 = Select(t=Plot_QSM_action."start updating" ("action"), s=w407, f=Plot_QSM_action."stop updating" ("action")) -> (s? t:f=w403:T23)
        n183 = Bundle By Name(cluster=T24 {"action"=enum."Update", "data"=variant} ("element"), "action"=w403) -> (w402:T24)
        n184 = Enqueue Element(queue=w409, element=w402) -> ()  [unwired: 2 in, 3 out]
        n185 = property on="visible sidebar?" class="Bool (strict)"("Val(Sgnl)"=w399) -> ()  [unwired: 2 in, 2 out]
        n186 = property on="Title Visible?" class="Bool (strict)"("Val(Sgnl)"=TRUE ("Value (Signaling)")) -> ()  [unwired: 2 in, 2 out]
        n187 = local write "Title"("Title" ("Title")) -> ()
        n188 = local write "visible?"(FALSE ("visible?")) -> ()
        n189 = local write "Erase Plot"(FALSE ("Clear Plots")) -> ()
        n190 = property on="Pane" class="Pane"("Origin"=T25 {"Horizontal"=0, "Vertical"=0}) -> ()  [unwired: 2 in, 2 out]
        n191 = local write "Splitter locked?"(TRUE ("Splitter locked?")) -> ()
        n192 = property on="dummy" class="Bool (strict)"("Val(Sgnl)"=TRUE ("Value (Signaling)")) -> ()  [unwired: 2 in, 2 out]
      }
      frame "start updating" {
        n193 = in-place {
          in-place-border: w414 -> [w418]
          n194 = in-place-cluster #4(w413) -> ("updating?"=w416:bool)
          n195 = case shown="False" w416 {
            tunnel: w418 -> [w420 _]
            frame False {
              n196 = Enqueue Element(queue=w420, element=T24 {"action"=enum."Update", "data"=variant}) -> ()  [unwired: 2 in, 3 out]
            }
            frame True {
            }
          }
          n197 = property on="visible?" class="Bool (strict)"("Val(Sgnl)"=TRUE ("Value (Signaling)")) -> ()  [unwired: 2 in, 2 out]
          n198 = in-place-cluster #4("updating?"=TRUE) -> (w412:T9)
        }
      }
      frame "stop updating" {
        n199 = Bundle By Name(cluster=w424, "updating?"=FALSE ("visible?")) -> (w422:T9)
        n200 = property on="visible?" class="Bool (strict)"("Val(Sgnl)"=FALSE ("Value (Signaling)")) -> ()  [unwired: 2 in, 2 out]
      }
      frame "Update" {
        n201 = Unbundle By Name(w425) -> ("updating?"=w428:bool)
        n202 = case shown="True" w428 {
          tunnel: w429 -> [_ w437]
          tunnel: w427 -> [_ w434]
          tunnel: w426 -> [_ w432]
          frame False {
          }
          frame True {
            n203 = Enqueue Element(queue=w434, element=T24 {"action"=enum."Update", "data"=variant}) -> ()  [unwired: 2 in, 3 out]
            n204 = local read "Time to Plot"() -> (w431:dbl)
            n205 = local read "top array"() -> (w448:T8[])
            n206 = Unbundle By Name(w437) -> ("Update rate (ms)"=w436:u32)
            n207 = call "has changed boolen - init first call.vi"("Boolean in"="Erase Plot") -> ("has changed?"=w442:bool, "Boolean out"=w443:bool)  [unwired: 9 in]
            n208 = call "has changed dbl first call.vi"("Numeric"=w431) -> ("has changed?"=w440:bool, "Numeric (dup)"=w445:dbl)  [unwired: 9 in]
            n209 = Compound Arithmetic op=AND(w443, w442) -> (w444:bool)
            n210 = Compound Arithmetic op=AND(invert w443, w442) -> (w441:bool)
            n211 = Or(x=w441, y=w440) -> (x .or. y?=w439:bool)
            n212 = Wait (ms)(milliseconds to wait=w436) -> ()  [unwired: 1 out]
            n213 = call "Get Oldest Time to Plot.vi"("reset? [F]"=w439, "History Length"=w445, "Clear Plot [F]"=w444) -> ("clear button active?"=w438:bool, "Oldest Time to Plot"=w435:dbl)  [unwired: 7 in]
            n214 = call "append horizontal lines to plot array.vi"("BluePlotHandle"=w432, "Oldest Time to Plot"=w435, "top array"=w448) -> ("Numerics"=→"Numerics":dbl[], "Plot data"=→"Plot":T26[])  [unwired: 7 in]
            n215 = local write "Erase Plot"(w438) -> ()
          }
        }
      }
      frame "Get Config" {
        n216 = Variant To Data(type=refnum<class "Promise.lvclass"> refnum ("Promise out"), Variant=w453) -> (data=w449:refnum<class "Promise.lvclass">, error out=w451:errorcluster)  [unwired: 1 in]
        n217 = case shown="No Error" w451 {
          tunnel: w454 -> [w458 _]
          tunnel: w449 -> [w457 _]
          frame No Error {
            n218 = call "Plot Load maker V2.vi"("Refs"=w458) -> ("error out"=w455:errorcluster, "Plot config"=w456:T1)  [unwired: 9 in]
            n219 = case shown="No Error" w455 {
              selector: w455 -> [_ w461]
              tunnel: w457 -> [w460 w462]
              tunnel: w456 -> [w459 _]
              frame No Error {
                n220 = call <vilib>:"Resolve with Result.vi"("Result"=w459, "Promise in"=w460) -> ()  [unwired: 9 in, 1 out]
              }
              frame Error {
                n221 = call <vilib>:"Resolve with Error.vi"("Result"=w461, "Promise in"=w462) -> ()  [unwired: 9 in, 1 out]
              }
            }
          }
          frame Error {
          }
        }
      }
      frame "Load Config" {
        n222 = Variant To Data(type=T1 {"plots"=[], "X-axis"={"Name Label.Text"="", "Style"=0, "Tick Colors:Minor Tick Color"=0, "Tick Colors:Tick Color"=0, "Marker Colors:Text Color"=0, "Grid Colors:Major Color"=0, "Grid Colors:Minor Color"=0, "Mapping Mode"=0, "Flipped"=FALSE, "Name Label.Visible"=FALSE, "Name Label.Text Colors:Text Color"=0, "Scale Fit"=0, "Editable"=FALSE, "Range:Maximum"=0.0, "Range:Minimum"=0.0, "Offset and Multiplier:Multiplier"=0.0, "Offset and Multiplier:Offset"=0.0, "Name Label.Font:Size"=0, "Marker.Font:Size"=0, "Uniform Marker Spacing?"=TRUE, "Format String"=""}, "Y-axes"=[], "General"={"Title"="", "Time to Plot"=1800.0, "Title.Visible"=FALSE, "Sidebar.Visible"=FALSE, "Plot Area:Colors:BG Color"=0}} ("Plot config"), Variant=w467) -> (data=w464:T1, error out=w466:errorcluster)  [unwired: 1 in]
        n223 = case shown="No Error" w466 {
          tunnel: w464 -> [w468 _]
          frame No Error {
            n224 = property on="Load Plot config" class="Clust (strict)"("Val(Sgnl)"=w468) -> ()  [unwired: 2 in, 2 out]
          }
          frame Error {
          }
        }
      }
      frame "Shutdown" {
        n225 = Release Queue(queue=w478) -> ()  [unwired: 2 in, 3 out]
        n226 = Unbundle By Name(w476) -> ("Meta LUT"=w475:refnum<data-value>)
        n227 = Delete Data Value Reference(data value reference=w475) -> ()  [unwired: 1 in, 2 out]
        n228 = Variant To Data(type=refnum<notifier> refnum ("notifier"), Variant=w471) -> (data=w469:refnum<notifier>, error out=w470:errorcluster)  [unwired: 1 in]
        n229 = call <vilib>:"Clear Errors.vi"("error in (no error)"=w470) -> ()  [unwired: 5 in, 2 out]
        n230 = property on="Shutdown" class="Bool (strict)"("Val(Sgnl)"=TRUE ("Value (Signaling)")) -> ()  [unwired: 2 in, 2 out]
      }
    }
  }
  n231 = flat-sequence {
    tunnel: w44 -> [_]
    tunnel: w43 -> [_]
    tunnel: w42 -> [_]
    tunnel: w5 -> [w480]
    frame #0 {
      # "shutdown"
      n232 = Send Notification(notification=TRUE, notifier=w480) -> ()  [unwired: 1 in, 2 out]
    }
  }
